vi "PathPlanner_Path_PositionDelta.vi"(9 "B":T1 {"Y" format="%14.3f"; "X" format="%14.3f"}, 11 "A":T1 {"Y" format="%14.3f"; "X" format="%14.3f"}) -> (3 "PosDelta":dbl)   [LabVIEW 2019, in "PathPlanner24.lvlib"]
doc: "Create a path f\nInputs:\n - \nOutputs:\n - PathPlanner Path -- The generated path"
uses:
  PathPlanner24.lvlib
  <vilib>/Rock Robotics/WPI/ThirdParty/JAS_Junk/TrajLib/TypeDef/TRANSLATION2D.ctl
  <vilib>/Rock Robotics/WPI/ThirdParty/JAS_Junk/TrajLib/Translation2d_Create.vi
  <vilib>/Rock Robotics/WPI/ThirdParty/JAS_Junk/TrajLib/Trajectory_Library.lvlib
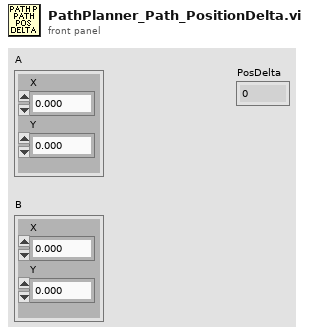
[diagram p1: front panel]
types:
  T1 = typedef "Trajectory_Library.lvlib/TRANSLATION2D.ctl" = cluster{"X":dbl, "Y":dbl}
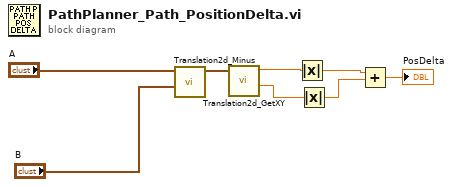
[diagram p0: block diagram]
diagram:
  n1 = call <vilib>:"Translation2d_Minus.vi"("other Translation"="B", "In Translation"="A") -> ("Out Translation"=w6:T1)  [unwired: 9 in]
  n2 = call <vilib>:"Translation2d_GetXY.vi"("In Translation"=w6) -> ("Y"=w4:dbl, "X"=w5:dbl)  [unwired: 9 in]
  n3 = Absolute Value(x=w5) -> (abs(x)=w3:dbl)
  n4 = Absolute Value(x=w4) -> (abs(x)=w2:dbl)
  n5 = Add(x=w3, y=w2) -> (x+y=→"PosDelta":dbl)
